vi "Speed_Sensor.vi"() -> ()   [LabVIEW 2013]
uses:
  <vilib>/Instr/_visa.llb/VISA Configure Serial Port (Instr).vi
panel:
  out "Gauge 2":dbl(knob) scale=0.0..50.0
  out "Gauge":dbl(knob) scale=0.0..3000.0
  out "Connection":bool
  in  "VISA resource name":refnum<visa-resource-name>
  in  "?":bool
  # "www.e3Help.in"
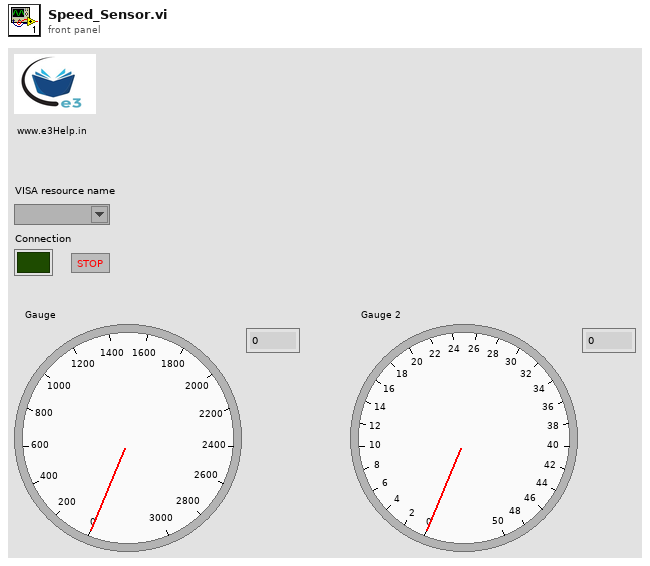
[diagram p1: front panel]
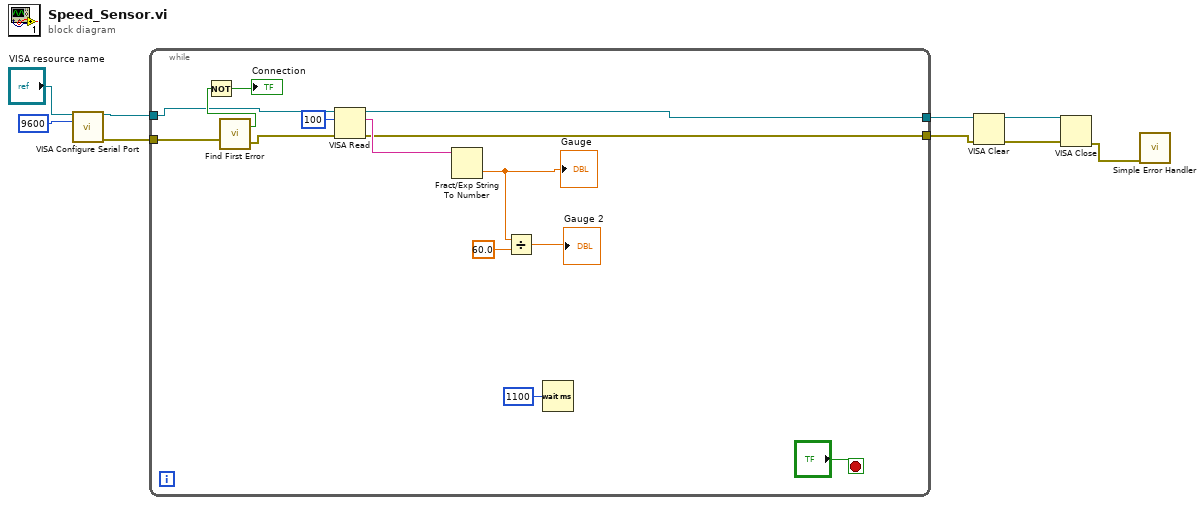
[diagram p0: block diagram]
diagram:
  n1 = call-poly "VISA Configure Serial Port"("VISA resource name"="VISA resource name", "baud rate (9600)"=u32 9600) -> ("VISA resource name out"=w7:refnum<visa-resource-name>, "error out"=w6:errorcluster)  [unwired: 12 in]
  n2 = while {
    tunnel: w7 -> [w18]
    tunnel: w6 -> [w22]
    tunnel: [w16] -> w2
    tunnel: [w14] -> w1
    stop <- "?" stop-if-true
    n3 = call <vilib>:"Find First Error.vi"("error in (no error)"=w22) -> ("error out"=w15:errorcluster, "error?"=w21:bool)  [unwired: 3 in]
    n4 = Not(x=w21) -> (.not. x?=→"Connection":bool)
    n5 = VISA Read(VISA resource name=w18, byte count=u32 100, error in (no error)=w15) -> (VISA resource name out=w16:refnum<visa-resource-name>, read buffer=w17:string, error out=w14:errorcluster)  [unwired: 1 out]
    n6 = Fract/Exp String To Number(string=w17) -> (number=w12:dbl)  [unwired: 3 in, 1 out]
    "Gauge" <- w12
    n7 = Divide(x=w12, y=60.0) -> (x/y=→"Gauge 2":dbl)
    n8 = Wait (ms)(milliseconds to wait=u32 1100) -> ()  [unwired: 1 out]
  }
  n9 = VISA Clear(VISA resource name=w2, error in (no error)=w1) -> (VISA resource name out=w5:refnum<visa-resource-name>, error out=w4:errorcluster)
  n10 = VISA Close(VISA resource name=w5, error in (no error)=w4) -> (error out=w3:errorcluster)
  n11 = call <vilib>:"Simple Error Handler.vi"("error in (no error)"=w3) -> ()  [unwired: 4 in, 5 out]
